vi "Arduino_HTTP_GetRequest.vi"(11 "Request string":string) -> (3 "body":string)   [LabVIEW 2017]
uses:
  <vilib>/httpClient/LabVIEWHTTPClient.lvlib
panel:
  out "headers":string
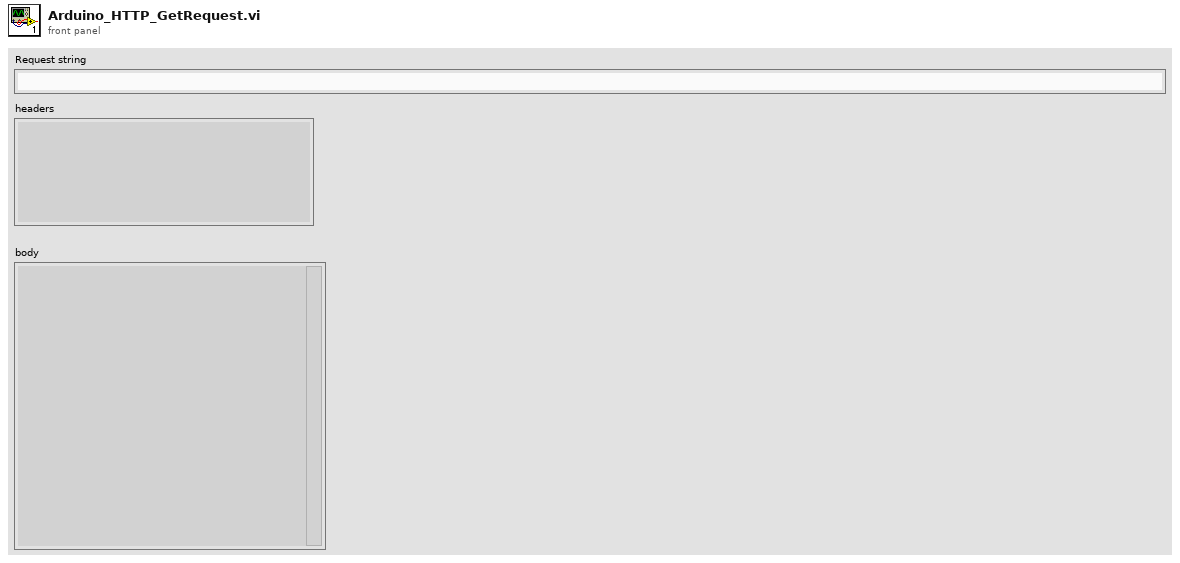
[diagram p1: front panel]
types:
  T1 = typedef "LabVIEWHTTPClient.lvlib/ClientHandle.ctl" = refnum<k1>
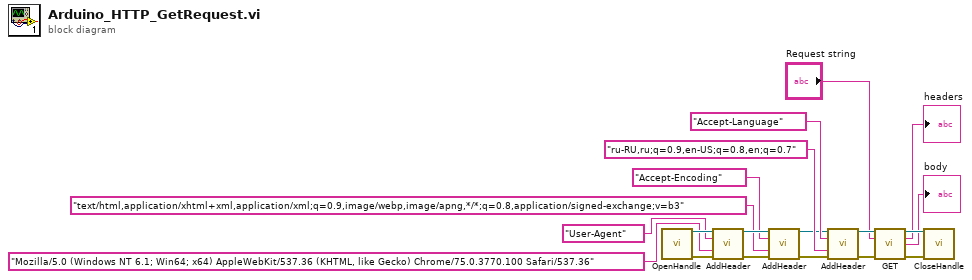
[diagram p0: block diagram]
diagram:
  n1 = call <vilib>:"OpenHandle.vi"() -> ("client handle out"=w19:T1, "error out"=w18:errorcluster)  [unwired: 14 in]
  n2 = call <vilib>:"AddHeader.vi"("client handle"=w19, "header"="User-Agent", "value"="Mozilla/5.0 (Windows NT 6.1; Win64; x64) AppleWebKit/537.36 (KHTML, like Gecko) Chrome/75.0.3770.100 Safari/537.36", "error in (no error)"=w18) -> ("client handle out"=w15:T1, "error out"=w14:errorcluster)  [unwired: 10 in]
  n3 = call <vilib>:"AddHeader.vi"("client handle"=w15, "header"="Accept-Encoding", "value"="text/html,application/xhtml+xml,application/xml;q=0.9,image/webp,image/apng,*/*;q=0.8,application/signed-exchange;v=b3", "error in (no error)"=w14) -> ("client handle out"=w9:T1, "error out"=w8:errorcluster)  [unwired: 10 in]
  n4 = call <vilib>:"AddHeader.vi"("client handle"=w9, "header"="Accept-Language", "value"="ru-RU,ru;q=0.9,en-US;q=0.8,en;q=0.7", "error in (no error)"=w8) -> ("client handle out"=w7:T1, "error out"=w6:errorcluster)  [unwired: 10 in]
  n5 = call <vilib>:"GET.vi"("client handle"=w7, "url"="Request string", "error in (no error)"=w6) -> ("client handle out"=w5:T1, "headers"=→"headers":string, "body"=→"body":string, "error out"=w4:errorcluster)  [unwired: 9 in]
  n6 = call <vilib>:"CloseHandle.vi"("client handle"=w5, "error in (no error)"=w4) -> ()  [unwired: 13 in, 1 out]
